vi "Is Encoded.vi"(11 "error in (no error)":errorcluster) -> (1 "Is Encoded":bool, 2 "offset past":i32, 3 "source":string)   [LabVIEW 2020, in "Multi Error Cluster.lvlib"]
uses:
  <vilib>/MultiError/TokenizeJSON/Multi Error Cluster.lvlib
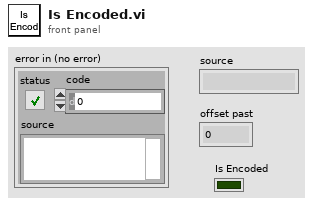
[diagram p1: front panel]
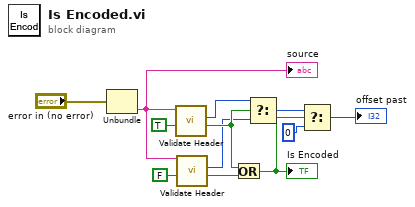
[diagram p0: block diagram]
diagram:
  n1 = Unbundle("error in (no error)") -> ("source"=w8:string)  [unwired: 2 out]
  "source" <- w8
  n2 = call <vilib>:"Validate Header.vi"("Single"=TRUE, "source"=w8) -> ("valid"=w11:bool, "offset past"=w10:i32)  [unwired: 8 in]
  n3 = call <vilib>:"Validate Header.vi"("Single"=FALSE, "source"=w8) -> ("valid"=w7:bool, "offset past"=w9:i32)  [unwired: 8 in]
  n4 = Or(x=w11, y=w7) -> (x .or. y?=w3:bool)
  "Is Encoded" <- w3
  n5 = Select(t=w10, s=w11, f=w9) -> (s? t:f=w2:i32)
  n6 = Select(t=w2, s=w3, f=0) -> (s? t:f=→"offset past":i32)
